vi "RampWhenSpeedingUp.vi"(10 "Ramp":dbl=1.0, 11 "Input":dbl(slide) scale=-1.0..1.0) -> (3 "Output":dbl(slide) scale=-1.0..1.0)   [LabVIEW 2016]
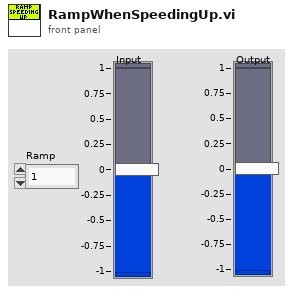
[diagram p1: front panel]
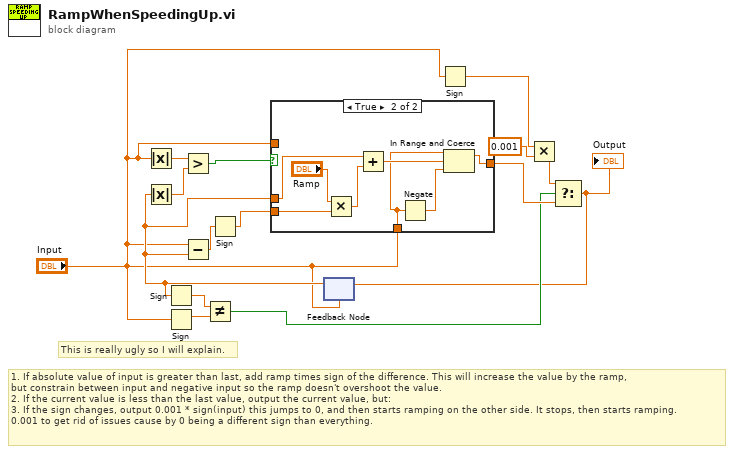
[diagram p0: block diagram]
diagram:
  # "1. If absolute value of input is greater than last, add ramp times sign of the difference. This will increase the value by the ramp,\nbut constrain between input and negative input so the ramp doesn't overshoot the value. \n2. If the current value is less than the last value, output the current value, but:\n3. If the sign changes, output 0.001 * sign(input) this jumps to 0, and then starts ramping on the other side. It stops, then starts ramping.\n0.001 to get rid of issues cause by 0 being a different sign than everything."
  # "This is really ugly so I will explain."
  n1 = Absolute Value(x="Input") -> (abs(x)=w15:dbl)
  n2 = Sign(1:"Input") -> (0:w9:dbl)
  n3 = feedback #1("Input") -> (w7:dbl)
  n4 = Absolute Value(x=w7) -> (abs(x)=w14:dbl)
  n5 = Sign(1:w7) -> (0:w10:dbl)
  n6 = Greater?(x=w15, y=w14) -> (0:w13:bool)
  n7 = Subtract(x="Input", y=w7) -> (x-y=w11:dbl)
  n8 = Not Equal?(x=w10, y=w9) -> (x != y?=w6:bool)
  n9 = Sign(1:w11) -> (0:w12:dbl)
  n10 = case shown="True" w13 {
    tunnel: [w16 w19] -> w8
    tunnel: w12 -> [_ w23]
    tunnel: w7 -> [_ w21]
    tunnel: "Input" -> [w16 _]
    tunnel: "Input" -> [_ w18]
    frame False {
    }
    frame True {
      n11 = Multiply(x="Ramp", y=w23) -> (x*y=w24:dbl)
      n12 = Add(x=w21, y=w24) -> (x+y=w20:dbl)
      n13 = Negate(x=w18) -> (-x=w17:dbl)
      n14 = In Range and Coerce(upper limit=w18, x=w20, lower limit=w17) -> (coerced(x)=w19:dbl)  [unwired: 1 out]
    }
  }
  n15 = Sign(1:"Input") -> (0:w3:dbl)
  n16 = Multiply(x=w3, y=0.001) -> (x*y=w5:dbl)
  n17 = Select(t=w5, s=w6, f=w8) -> (s? t:f=w2:dbl)
  "Output" <- w2
  n18 = feedback-in #1(w2) -> ()
